vi "Stop Core.vi"(10 "final error code":i32, 11 "Actor_Log in":refnum<class "Actor_EventStart.lvclass">) -> (3 "Actor_Log out":refnum<class "Actor_EventStart.lvclass">)   [LabVIEW 2020, in "Library Core.lvlib" / "Actor_EventStart.lvlib" / "Actor_EventStart.lvclass"]
doc: "(<B>Filename</B>: Actor Framework.lvlib:Actor.lvclass:Stop Core.vi)\n\nDefines what the actor does before it stops. Use the <B>final error code</B> input to determine whether the actor shut down in response to an error.\n\nBy default, this method does nothing. A descendant class may override it to define behavior, such as shutting down any processes the actor initiated in its override of the Actor Core method."
uses:
  Actor_EventStart.lvclass
  Actor_EventStart.lvclass/Actor_EventStart.ctl
  <vilib>/ActorFramework/Actor/Actor.lvclass
  Commun VI/Library Commun.lvlib
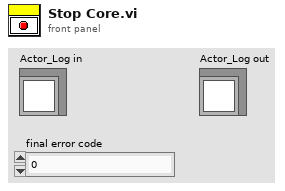
[diagram p1: front panel]
types:
  T1 = enum16{"Init", "Add Actor", "Delete Actor", "Get Actor Queue", "Get Log Actor Queue", "List all actors"}
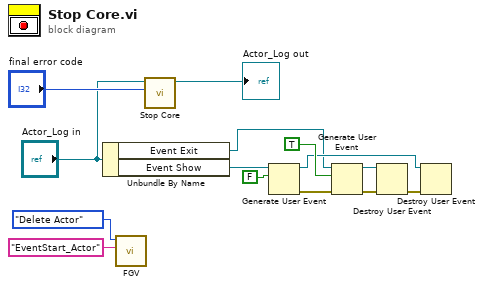
[diagram p0: block diagram]
diagram:
  n1 = Unbundle By Name("Actor_Log in") -> ("Event Exit"=w1:refnum<user-event>, "Event Show"=w7:refnum<user-event>)
  n2 = call "FGV.vi"("Actor name"="EventStart_Actor", "Action"=T1."Delete Actor") -> ()  [unwired: 7 in, 3 out]
  n3 = call-parent "Stop Core.vi"("final error code"="final error code", "Actor in"="Actor_Log in") -> ("Actor out"=→"Actor_Log out":refnum<class "Actor_EventStart.lvclass">)  [unwired: 9 in]
  n4 = Generate User Event(user event=w7, event data cluster=FALSE ("event data")) -> (user event out=w2:refnum<user-event>, error out=w6:errorcluster)  [unwired: 2 in]
  n5 = Generate User Event(user event=w1, event data cluster=TRUE ("event data"), error in=w6) -> (user event out=w4:refnum<user-event>, error out=w5:errorcluster)  [unwired: 1 in]
  n6 = Destroy User Event(user event=w4, error in=w5) -> (error out=w3:errorcluster)
  n7 = Destroy User Event(user event=w2, error in=w3) -> ()  [unwired: 1 out]
